vi "set voltage.vi"(8 "error in (no error)":errorcluster, 10 "Voltage":dbl, 11 "PSP-603 in":refnum<class "PSP-603.lvclass">) -> (0 "error out":errorcluster, 3 "PSP-603 out":refnum<class "PSP-603.lvclass">)   [LabVIEW 2025, in "Power Supply.lvlib" / "PSP-603.lvclass"]
uses:
  PSP-603.lvclass
  PSP-603.lvclass/PSP-603.ctl
panel:
  out "concatenated string":string
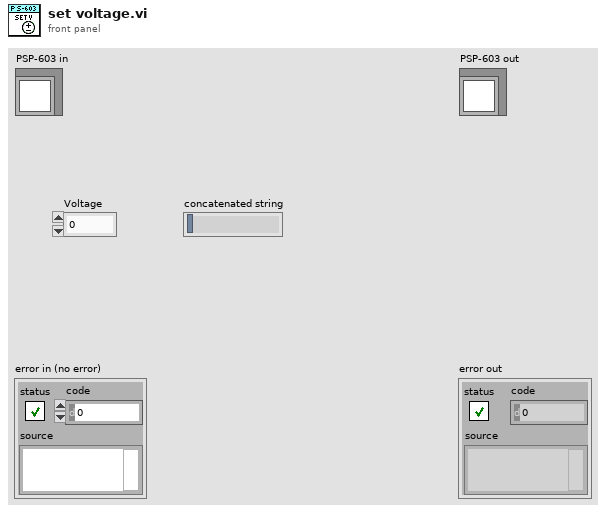
[diagram p1: front panel]
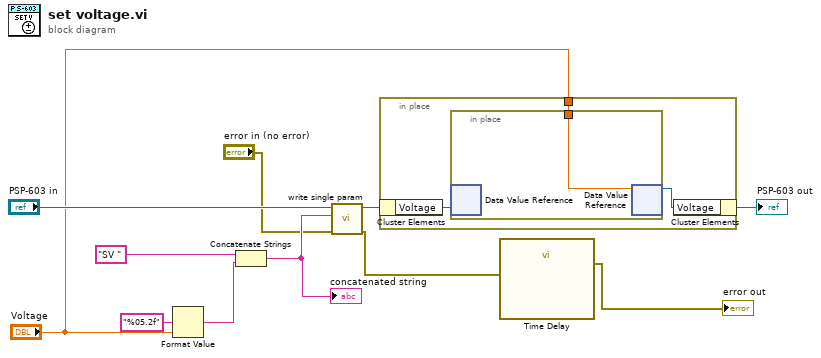
[diagram p0: block diagram]
diagram:
  n1 = Format Value(format string="%05.2f", value (0)="Voltage") -> (output string=w8:string)  [unwired: 1 in]
  n2 = Concatenate Strings("SV ", w8) -> (w7:string)
  "concatenated string" <- w7
  n3 = call-dynamic "write single param.vi"("error in (no error)"="error in (no error)", "string"=w7, "PSP-603 in"="PSP-603 in") -> ("error out"=w5:errorcluster, "PSP-603 out"=w3:refnum<class "PSP-603.lvclass">)  [unwired: 7 in]
  n4 = in-place {
    in-place-border: "Voltage" -> [w12]
    n5 = in-place-cluster #1(w3) -> ("Voltage"=w14:refnum<data-value>)
    n6 = in-place {
      in-place-border: w12 -> [w15]
      n7 = in-place-dvr #2(w14) -> ()  [unwired: 2 out]
      n8 = in-place-dvr #2(w15) -> (w13:refnum<data-value>)  [unwired: 1 out]
    }
    n9 = in-place-cluster #1("Voltage"=w13) -> (→"PSP-603 out":refnum<class "PSP-603.lvclass">)
  }
  n10 = call "Time Delay"("error in (no error)"=w5) -> ("error out"=→"error out":errorcluster)  [unwired: 10 in]
